vi "amplitude modulation.vi"() -> ()   [LabVIEW 2025]
uses:
  <vilib>/express/express analysis/Spectral/Block/exnSpectralBlock spectral measurements RMS poly.vi
  <vilib>/express/express analysis/Spectral/Block/exnSpectralBlock spectral measurements RMS DDT.vi
  <vilib>/express/express analysis/Spectral/XNode/ExpressSpectralMeasurementsBlockNode.xnode
panel:
  out "FFT RMS":dynamicdata(graph)
  out "Filtered Signal":dynamicdata(graph)
  out "modulated signal":dynamicdata(graph)
  in  "Amplitude":dbl=1.0
  out "carrier signal":dynamicdata(graph)
  out "message signal Graph":dynamicdata(graph)
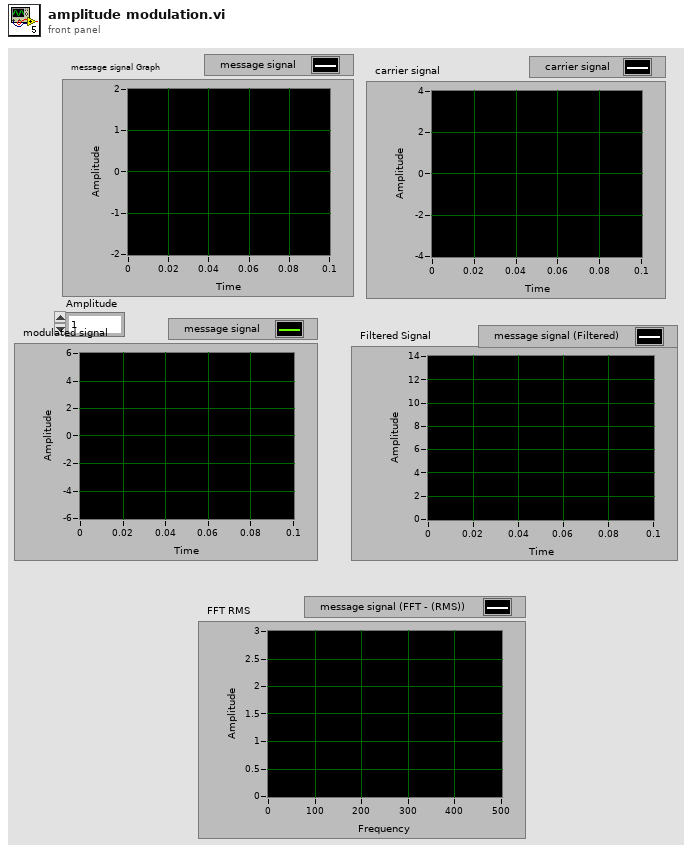
[diagram p1: front panel]
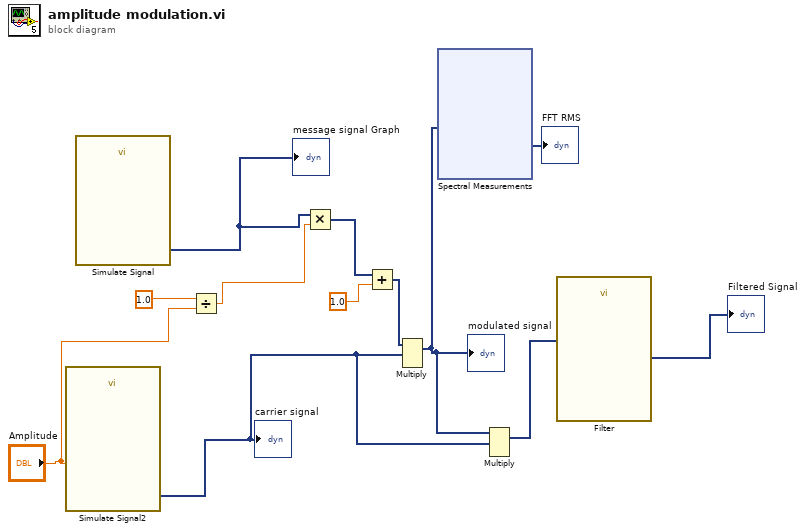
[diagram p0: block diagram]
diagram:
  n1 = call "Simulate Signal2"("Amplitude"="Amplitude") -> ("carrier signal"=w2:dynamicdata)  [unwired: 13 in, 1 out]
  "carrier signal" <- w2
  n2 = call "Simulate Signal"() -> ("message signal"=w12:dynamicdata)  [unwired: 14 in, 1 out]
  "message signal Graph" <- w12
  n3 = Divide(x=1.0 ("y"), y="Amplitude") -> (x/y=w11:dbl)
  n4 = Multiply(x=w12, y=w11) -> (x*y=w10:dynamicdata)
  n5 = Add(x=w10, y=1.0) -> (x+y=w6:dynamicdata)
  n6 = Multiply(1:w2, 2:w6) -> (0:w5:dynamicdata)  [unwired: 1 in, 1 out]
  "modulated signal" <- w5
  n7 = xnode "Spectral Measurements"("Signals"=w5) -> ("FFT - (RMS)"=→"FFT RMS":dynamicdata)  [unwired: 1 in, 2 out]
  n8 = Multiply(1:w2, 2:w5) -> (0:w1:dynamicdata)  [unwired: 1 in, 1 out]
  n9 = call "Filter"("Signal"=w1) -> ("Filtered Signal"=→"Filtered Signal":dynamicdata)  [unwired: 9 in, 1 out]
